vi "Newport_PM_Range_Select.vi"(6 "RANGE SEL":i32 min=0 max=7 step=1, 7 "DUT Count":i32=1 min=1 max=8 step=1, 8 "Error In":errorcluster, 11 "Reference In":refnum<k24>) -> (0 "Error Out":errorcluster, 1 "Query Response":string, 2 "Range Setting Confirmed":bool, 3 "Reference Out":refnum<k24>)   [LabVIEW 2017]
uses:
  C:/Program Files (x86)/Newport/Newport USB Driver/Bin/UsbDllWrap.dll
  Program Files (x86)/Newport/Newport USB Driver/Bin/UsbDllWrap.dll
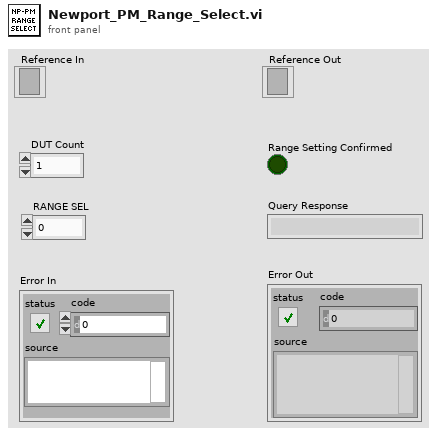
[diagram p1: front panel]
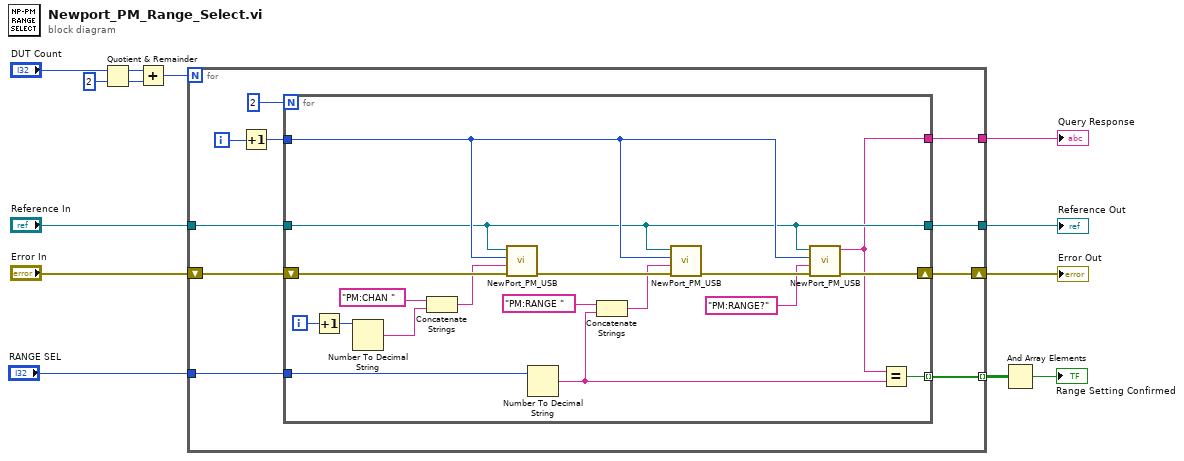
[diagram p0: block diagram]
diagram:
  n1 = Quotient & Remainder(x="DUT Count", y=2) -> (x-y*floor(x/y)=w7:i32, floor(x/y)=w8:i32)
  n2 = Add(x=w7, y=w8) -> (x+y=w6:i32)
  n3 = for {
    N: w6 -> [_]
    tunnel: "Reference In" -> [w19]
    shift-right: [w23] -> w12
    shift-left: "Error In" -> [w17]
    tunnel: [w21] -> w5 mode=indexing
    tunnel: [w20] -> w3
    tunnel: [w15] -> w2
    tunnel: "RANGE SEL" -> [w14]
    i -> [w22]
    n4 = Increment(x=w22) -> (x+1=w18:i32)
    n5 = for {
      N: 2 -> [_]
      tunnel: [w38] -> w21 mode=indexing
      tunnel: [w25] -> w20
      tunnel: w19 -> [w31]
      tunnel: w18 -> [w37]
      shift-right: [w40] -> w23
      shift-left: w17 -> [w36]
      tunnel: [w31] -> w15
      tunnel: w14 -> [w27]
      i -> [w30]
      n6 = Increment(x=w30) -> (x+1=w29:i32)
      n7 = Number To Decimal String(number=w29) -> (decimal integer string=w32:string)  [unwired: 1 in]
      n8 = Concatenate Strings("PM:CHAN " ("PM:CMD_QUERY In"), w32) -> (w33:string)
      n9 = call "NewPort_PM_USB.vi"("error in"=w36, "PM:CMD_QUERY In"=w33, "USB Address"=w37, "reference"=w31) -> ("error out"=w35:errorcluster)  [unwired: 5 in, 2 out]
      n10 = Number To Decimal String(number=w27) -> (decimal integer string=w24:string)  [unwired: 1 in]
      n11 = Concatenate Strings("PM:RANGE " ("PM:CMD_QUERY In"), w24) -> (w26:string)
      n12 = call "NewPort_PM_USB.vi"("error in"=w35, "PM:CMD_QUERY In"=w26, "USB Address"=w37, "reference"=w31) -> ("error out"=w41:errorcluster)  [unwired: 5 in, 2 out]
      n13 = call "NewPort_PM_USB.vi"("error in"=w41, "PM:CMD_QUERY In"="PM:RANGE?", "USB Address"=w37, "reference"=w31) -> ("error out"=w40:errorcluster, "Query-String\nfrom Read Buffer\nComplete Info"=w25:string)  [unwired: 5 in, 1 out]
      n14 = Equal?(x=w25, y=w24) -> (x = y?=w38:bool)
    }
  }
  "Error Out" <- w12
  "Query Response" <- w3
  "Reference Out" <- w2
  n15 = And Array Elements(Boolean array=w5) -> (logical AND=→"Range Setting Confirmed":bool)
